vi "Fresnel.vi"() -> ()   [LabVIEW 2019]
uses:
  <vilib>/imath/engines/lvmath2/RunTimeEngine/RangeToken/NIMS_Range.vi
  <instcachedir>/0/NIMS_Range_0856D726B6B24596B614846B21C682A9.lvgen/NIMS_Range_0856D726B6B24596B614846B21C682A9_001.vi
  <vilib>/imath/engines/lvmath2/RunTimeEngine/BuiltInFunctions/meshgrid2d/NIMS_meshgrid2d(V,V).vi
  <instcachedir>/0/NIMS_meshgrid2d(V,V)_3733343E1C554A708015CFB0432C6A59.lvgen/NIMS_meshgrid2d(V,V)_3733343E1C554A708015CFB0432C6A59_005.vi
  <vilib>/imath/engines/lvmath2/RunTimeEngine/ErrorHandling/NIMS_Create Error From Enums.vi
  <vilib>/imath/engines/lvmath2/RunTimeEngine/ArithmeticOperatorToken/NIMS_ArithmeticOperator_plus.vi
  <instcachedir>/0/NIMS_ArithmeticOperator_plus_A857F7369B7D4E138264023AAAB8243E.lvgen/NIMS_ArithmeticOperator_plus_A857F7369B7D4E138264023AAAB8243E_003.vi
  <vilib>/imath/engines/lvmath2/RunTimeEngine/BuiltInFunctions/mod/NIMS_mod_no_size_check.vi
  <instcachedir>/0/NIMS_mod_no_size_check_5393E3382FD241D281EEB71DA286C65B.lvgen/NIMS_mod_no_size_check_5393E3382FD241D281EEB71DA286C65B_004.vi
  <vilib>/imathl/engines/lvmath/Functions/Error Handling/Create Error.vi
  <vilib>/imath/engines/lvmath2/RunTimeEngine/BuiltInFunctions/uint16/NIMS_uint16(real).vi
  <instcachedir>/0/NIMS_uint16(real)_2A12B316DA9F4E3DA4FBB9443F5FDC71.lvgen/NIMS_uint16(real)_2A12B316DA9F4E3DA4FBB9443F5FDC71_001.vi
  <vilib>/imath/engines/lvmath2/RunTimeEngine/NodeEndStatement/NIMS_NodeEndStatement_Output.vi
  <instcachedir>/0/NIMS_NodeEndStatement_Output_53EC0D466D134D7ABD903AC30B43404B.lvgen/NIMS_NodeEndStatement_Output_53EC0D466D134D7ABD903AC30B43404B_010.vi
  <vilib>/imath/engines/lvmath2/RunTimeEngine/ErrorHandling/NIMS_Finalize Error.vi
panel:
  out "Phase SLM":T1(plugin-control)
  in  "f":dbl=1.0
  in  "Stop":bool
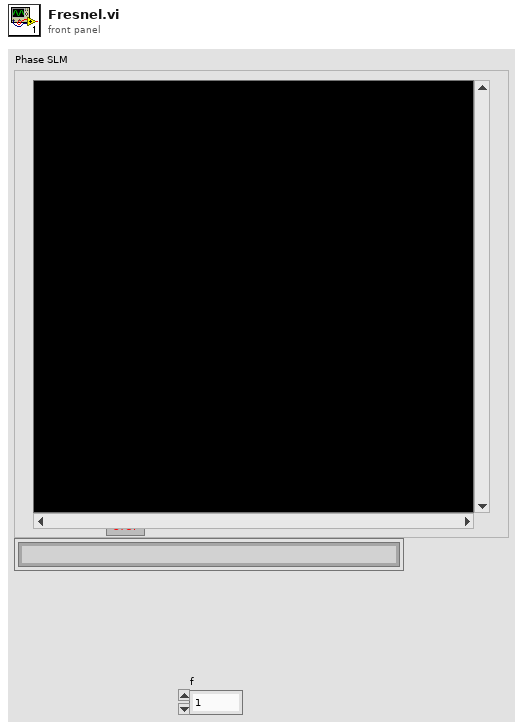
[diagram p1: front panel]
types:
  T1 = typedef "IMAQ Image.ctl" = refnum<image>
  T2 = typedef "Image Type" = u32
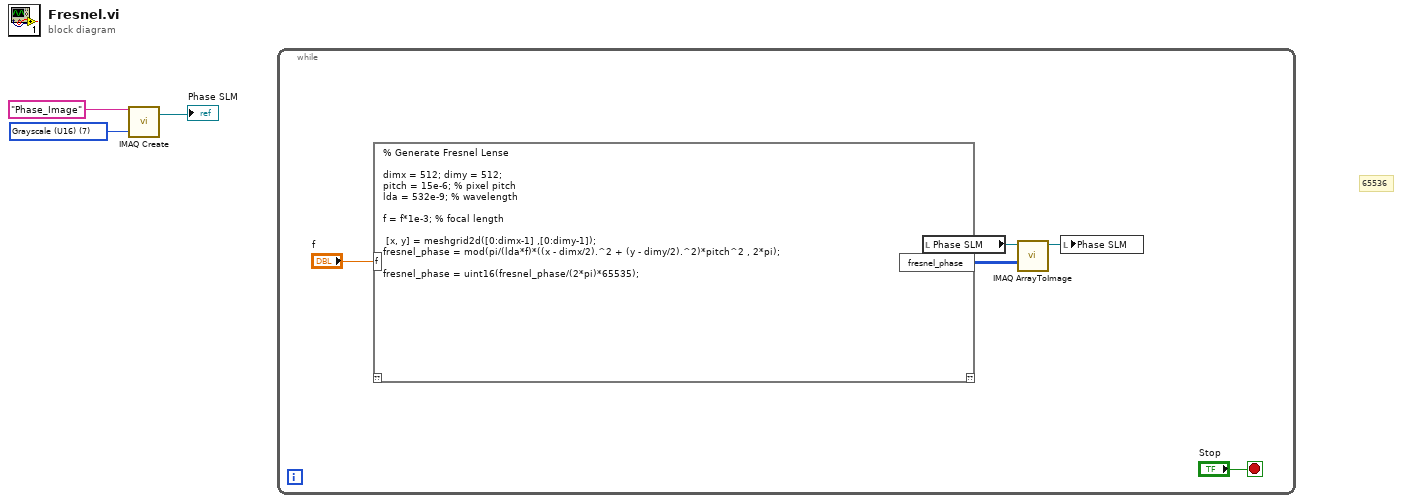
[diagram p0: block diagram]
diagram:
  w2 = T2 7 items=["Grayscale (U8)", "Grayscale (I16)", "Grayscale (SGL)", "Complex (CSG)", "RGB (U32)", "HSL (U32)", "RGB (U64)", "Grayscale (U16)"] ("Image Type")
  # "65536"
  n1 = call "IMAQ Create"("Image Name"="Phase_Image", "Image Type"=w2) -> ("New Image"=→"Phase SLM":T1)  [unwired: 3 in, 1 out]
  n2 = while {
    stop <- "Stop" stop-if-true
    n3 = mathscript code="% Generate Fresnel Lense\n\ndimx = 512; dimy = 512;\npitch = 15e-6; % pixel pitch\nlda = 532e-9; % wavelength\n\nf = f*1e-3; % focal length\n\n [x, y] = meshgrid2d([0:dimx-1] ,[0:dimy-1]);\nfresnel_phase = mod(pi/(lda*f)*((x - dimx/2).^2 + (y - dimy/2).^2)*pitch^2 , 2*pi);\n\nfresnel_phase = uint16(fresnel_phase/(2*pi)*65535);"("f"="f") -> ("fresnel_phase"=w6:u16[][])  [unwired: 1 in, 1 out]
    n4 = local read "Phase SLM"() -> (w5:T1)
    n5 = call "IMAQ ArrayToImage"("Image Pixels (U16)"=w6, "Image"=w5) -> ("Image Out"=w4:T1)  [unwired: 8 in, 1 out]
    n6 = local write "Phase SLM"(w4) -> ()
  }
